vi "PhotonPipelineMetadata_Pack.vi"(11 "PhotonPipelineMetadata":T1={"CaptureTimestampMicros"=-1, "PublishTimestampMicros"=-1, "SequenceID"=-1, "TimeSinceLastPong"=9999999999}) -> (3 "Packet_RawData":u8[](array[numeric]))   [LabVIEW 2019, in "PhotonVisionLib.lvlib"]
doc: "Convert a PipelineMetadat cluster to a Packet array of bytes ready for writing to a Network Table variable.\n\nInputs:\n - PipelineMetadata -- PipelineMetadata cluster.\n\nOutputs:\n - Pacet_RawData -- Byte array containing the encoded PipelineResult."
uses:
  PhotonVisionLib.lvlib
  TypeDef/PhotonPipelineMetadataType.ctl
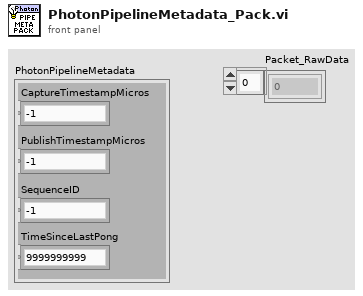
[diagram p1: front panel]
types:
  T1 = typedef "PhotonVisionLib.lvlib/PhotonPipelineMetadataType.ctl" = cluster{"CaptureTimestampMicros":i64, "PublishTimestampMicros":i64, "SequenceID":i64, "TimeSinceLastPong":i64}
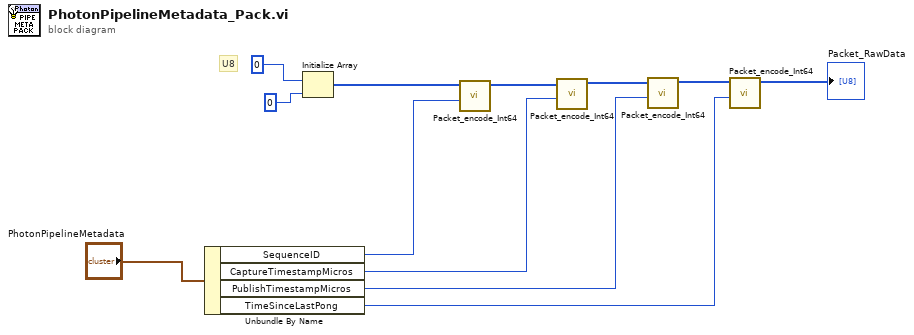
[diagram p0: block diagram]
diagram:
  # "U8"
  n1 = Unbundle By Name("PhotonPipelineMetadata") -> ("SequenceID"=w8:i64, "CaptureTimestampMicros"=w3:i64, "PublishTimestampMicros"=w2:i64, "TimeSinceLastPong"=w1:i64)
  n2 = Initialize Array(u8 0 ("element"), 0 ("dimension size")) -> (w9:u8[])
  n3 = call "Packet_encode_Int64.vi"("Int64_Value"=w8, "RawData In"=w9) -> ("RawData Out"=w7:u8[])  [unwired: 9 in]
  n4 = call "Packet_encode_Int64.vi"("Int64_Value"=w3, "RawData In"=w7) -> ("RawData Out"=w6:u8[])  [unwired: 9 in]
  n5 = call "Packet_encode_Int64.vi"("Int64_Value"=w2, "RawData In"=w6) -> ("RawData Out"=w5:u8[])  [unwired: 9 in]
  n6 = call "Packet_encode_Int64.vi"("Int64_Value"=w1, "RawData In"=w5) -> ("RawData Out"=→"Packet_RawData":u8[])  [unwired: 9 in]
